vi "Pomiar charakterystyk tranzystora.vi"() -> ()   [LabVIEW 2023]
uses:
  states ilosc charakterystyk type def.ctl
  Typedef.ctl
  Open_device_2018.llb/Select_Instr.ctl
  <vilib>/Analysis/1siggen.llb/Ramp Pattern by Samples.vi
  <vilib>/Utility/file.llb/Write Delimited Spreadsheet (DBL).vi
  <vilib>/Analysis/NI_AALBase.lvlib
panel:
  in  "Zatwierdz":bool
  out "Moc 3":dbl[](array[numeric])
  out "Ic 3":dbl[](array[numeric])
  out "Uce 3":dbl[](array[numeric])
  out "XY Graph":cluster{dbl[], dbl[]}[](graph)=[{[1.0, 2.0, 4.0], [2.0, 1.0, 0.0]}, {[0.5, 1.5, 3.5], [3.0, 4.0, 2.0]}]
  out "Ic 2":dbl[](array[numeric])
  out "Moc 2":dbl[](array[numeric])
  out "Uce 2":dbl[](array[numeric])
  out "Samples 3":dbl[](array[numeric])
  out "Samples 2":dbl[](array[numeric])
  out "Samples":dbl[](array[numeric])
  in  "Maksymalne napiecie zasilania 3":i32=30
  in  "Maksymalne napiecie zasilania 2":i32=30
  in  "Maksymalne napiecie zasilania":i32=30
  in  "Ilosc punktow pomiarowych 3":i32=60
  in  "Ilosc punktow pomiarowych 2":i32=60
  in  "Ilosc punktow pomiarowych":i32=60
  out "Moc":dbl[](array[numeric])
  out "Uce":dbl[](array[numeric])
  out "Ic":dbl[](array[numeric])
  in  "Wybor operacji po pomiarze":enum16{"Exit", "Eksportuj do pliku"}(ring)
  in  "Maksymalna moc tranzystora 3":dbl(knob) scale=0.0..0.8
  in  "Maksymalna moc tranzystora 2":dbl(knob) scale=0.0..0.8
  in  "OK":bool
  out "Dzialanie programu":string
  in  "Zakoncz program":bool
  in  "Maksymalna moc tranzystora":dbl(knob) scale=0.0..0.8
  in  "Prad bazy 3":enum16{"100uA", "200uA", "300uA"}(ring)=enum."300uA"
  in  "Prad bazy 2":enum16{"100uA", "200uA", "300uA"}(ring)=enum."200uA"
  in  "Prad bazy":enum16{"100uA", "200uA", "300uA"}(ring)
  in  "Ilosc charakterystyk":T1
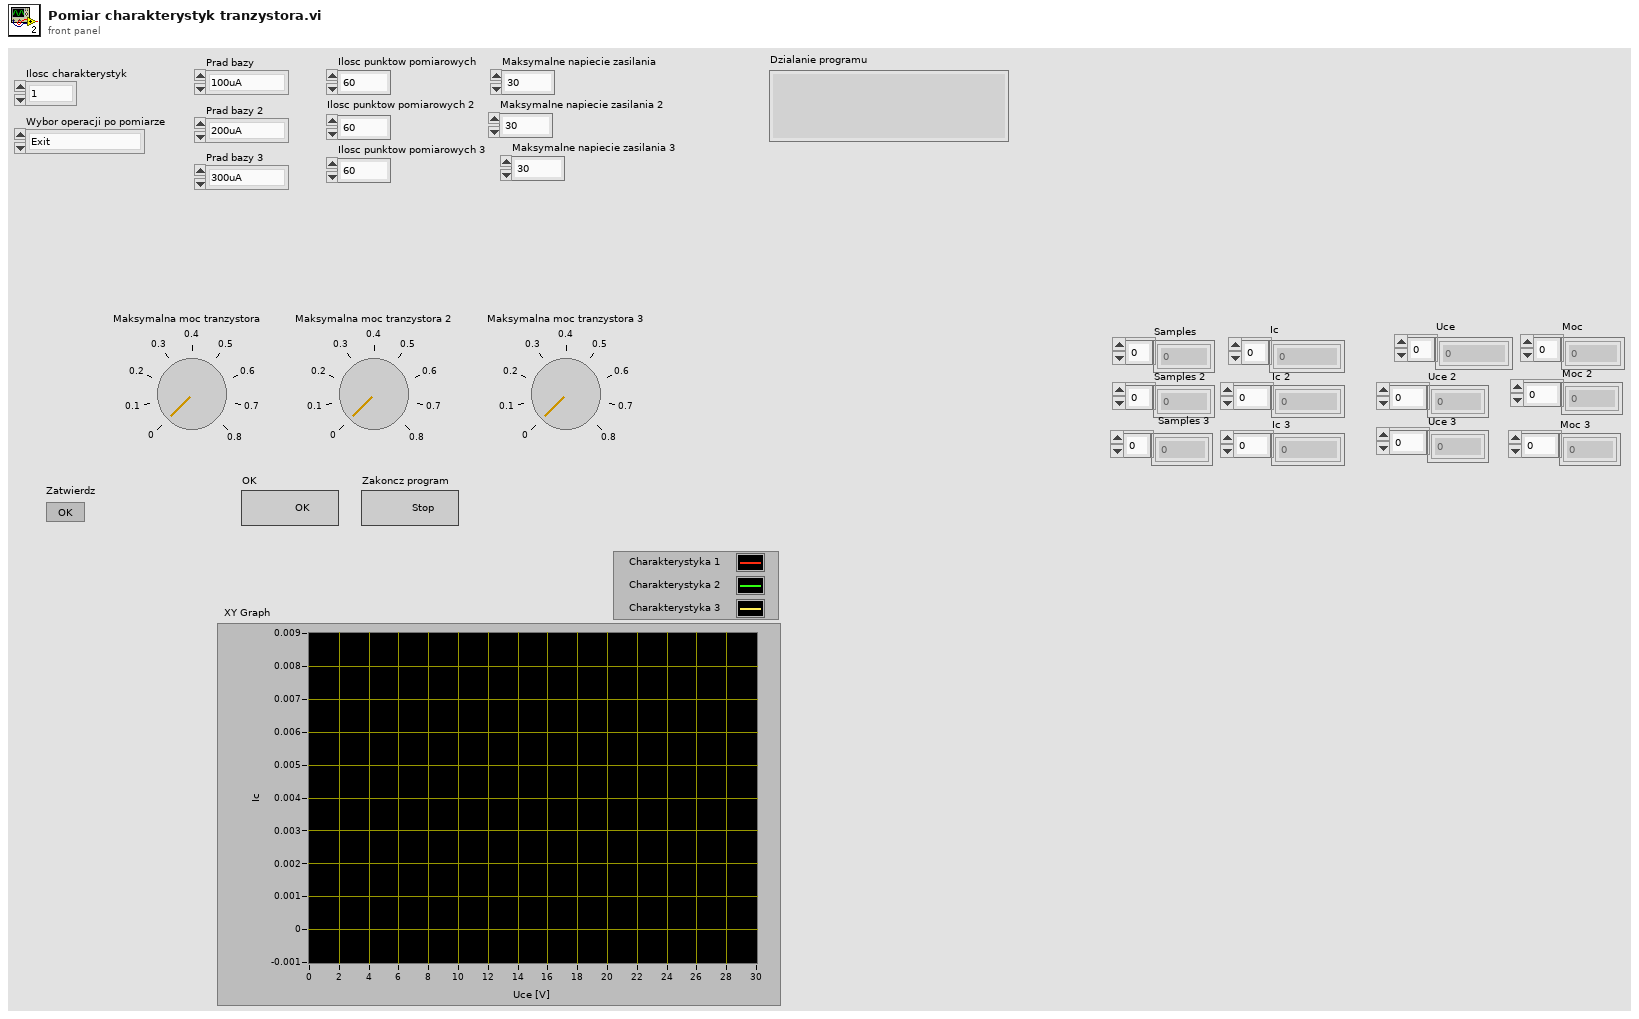
[diagram p1: front panel]
types:
  T1 = typedef "states ilosc charakterystyk type def.ctl" = enum16{"1", "2", "3"}
  T2 = typedef "Typedef.ctl" = enum16{"init", "idle", "Pomiar", "Po pomiarze", "Eksportuj do pliku", "Exit"}
  T3 = typedef "Select_Instr.ctl" = string
  T4 = cluster{"Zasilacz BM572":refnum<visa-resource-name>, "Komutator L201":refnum<visa-resource-name>, "Multimetr V553":refnum<visa-resource-name>}
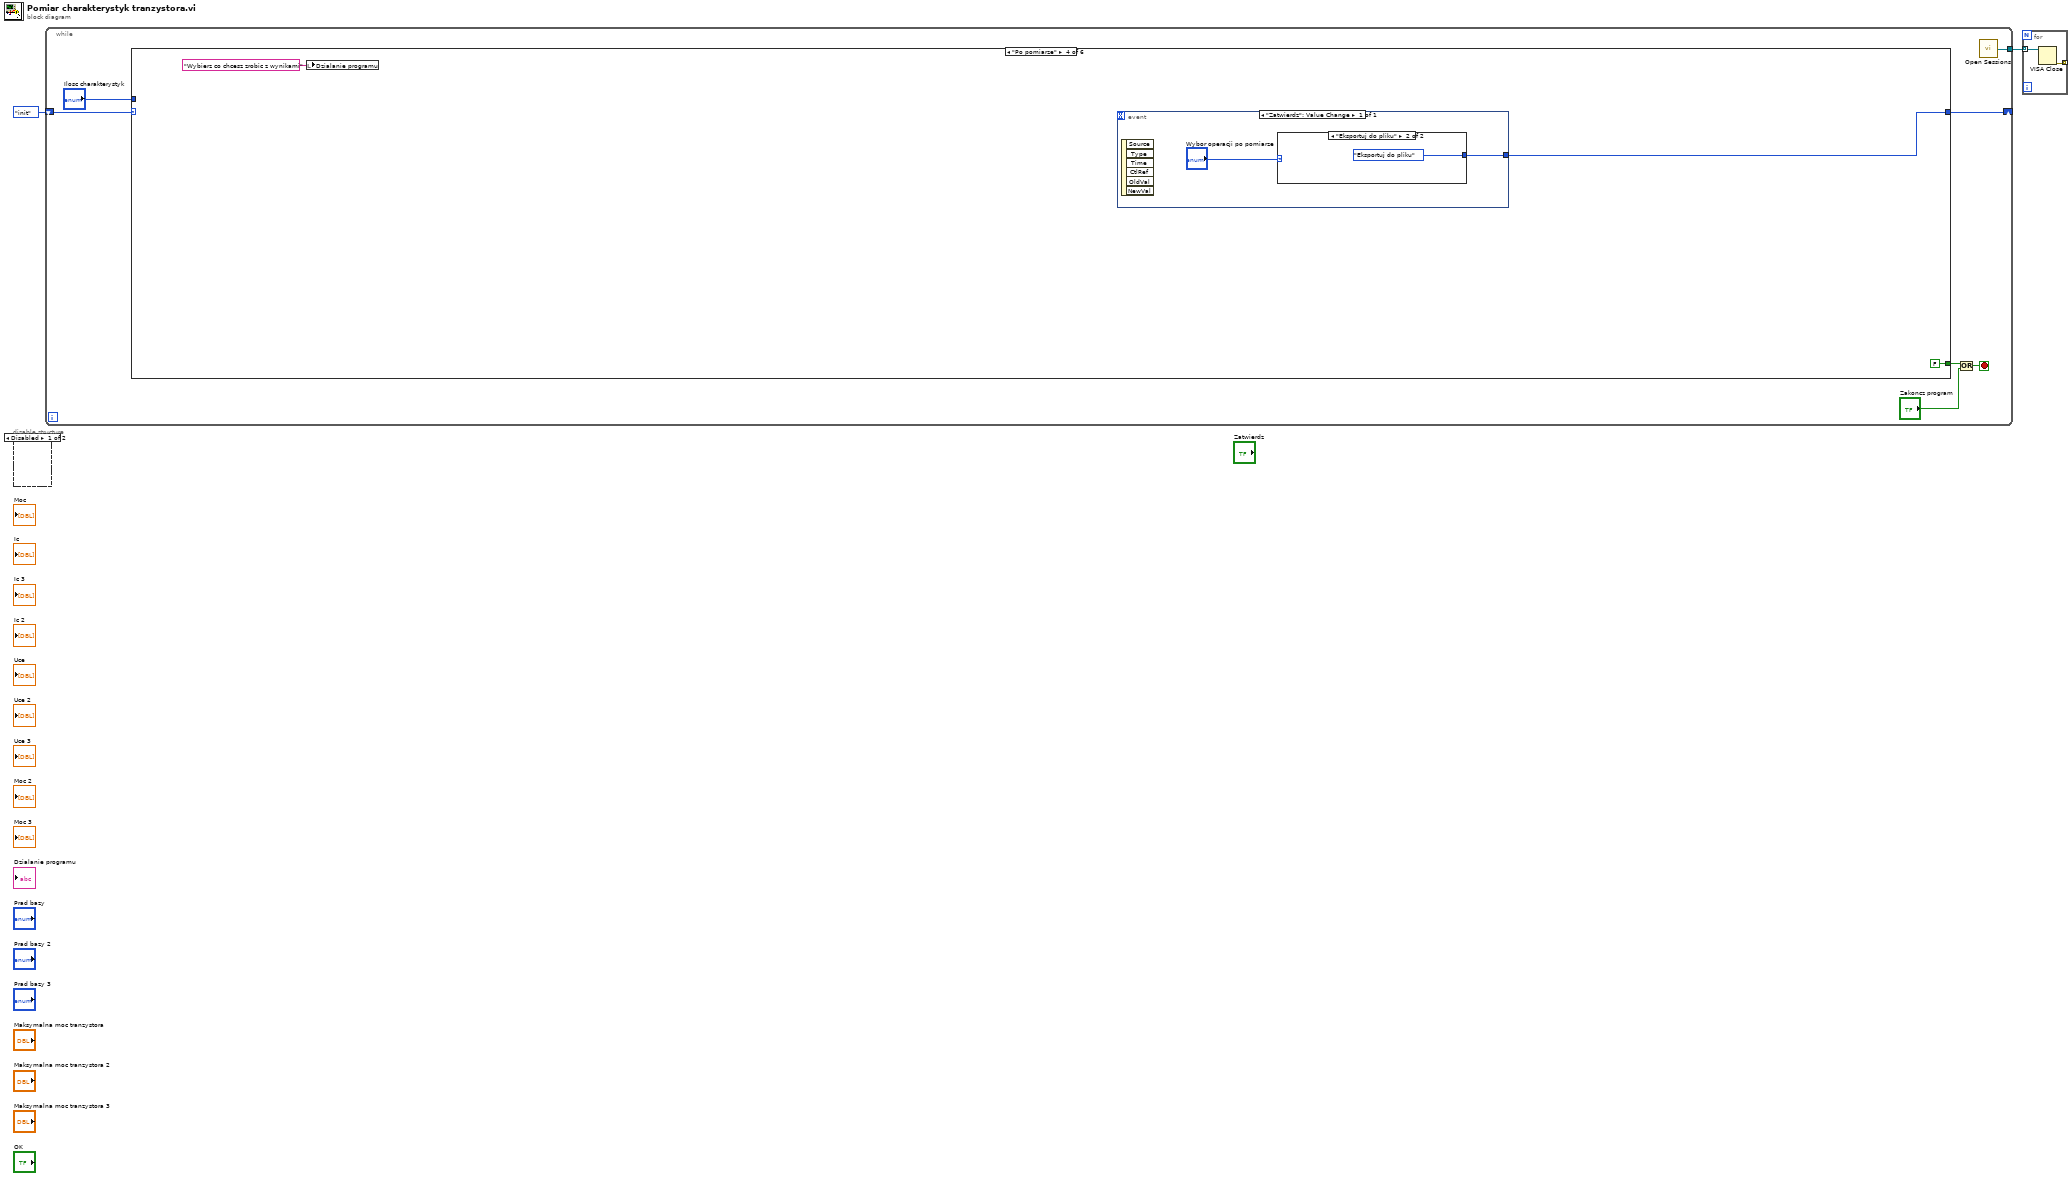
[diagram p0: block diagram]
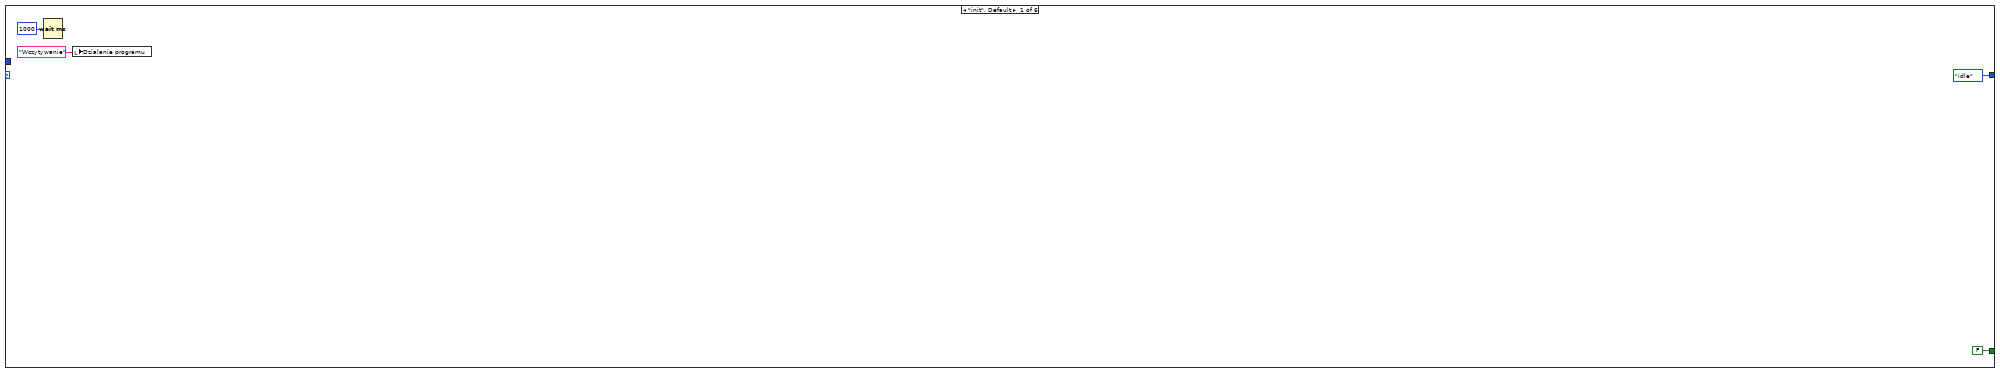
[diagram p3: hidden frame]
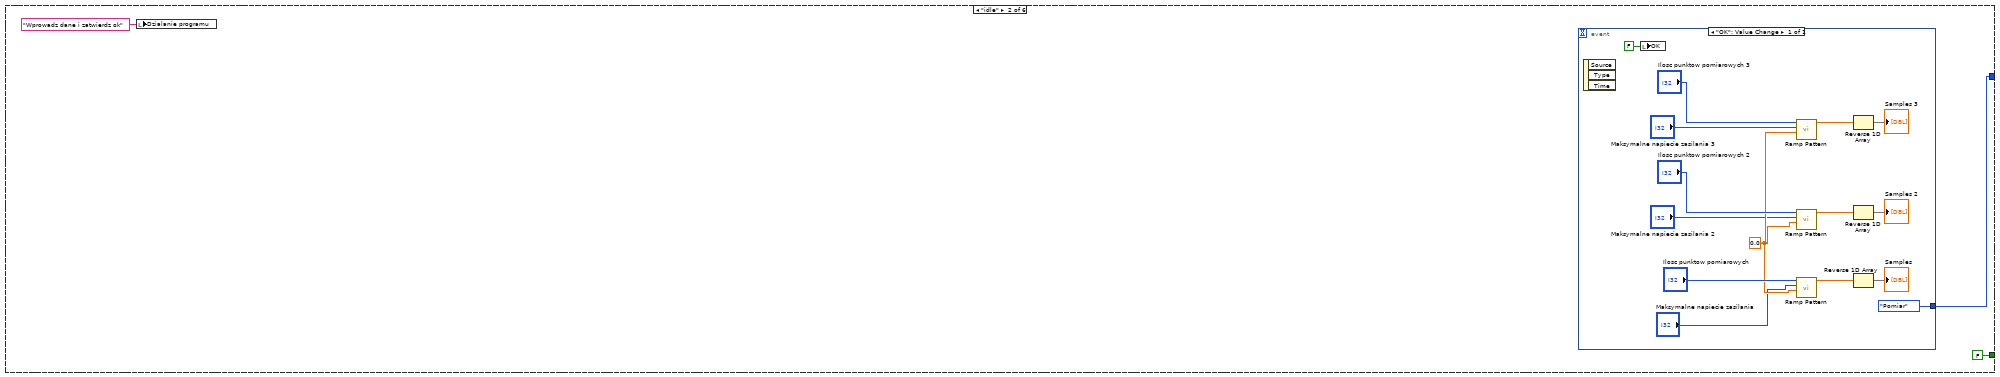
[diagram p4: hidden frame]
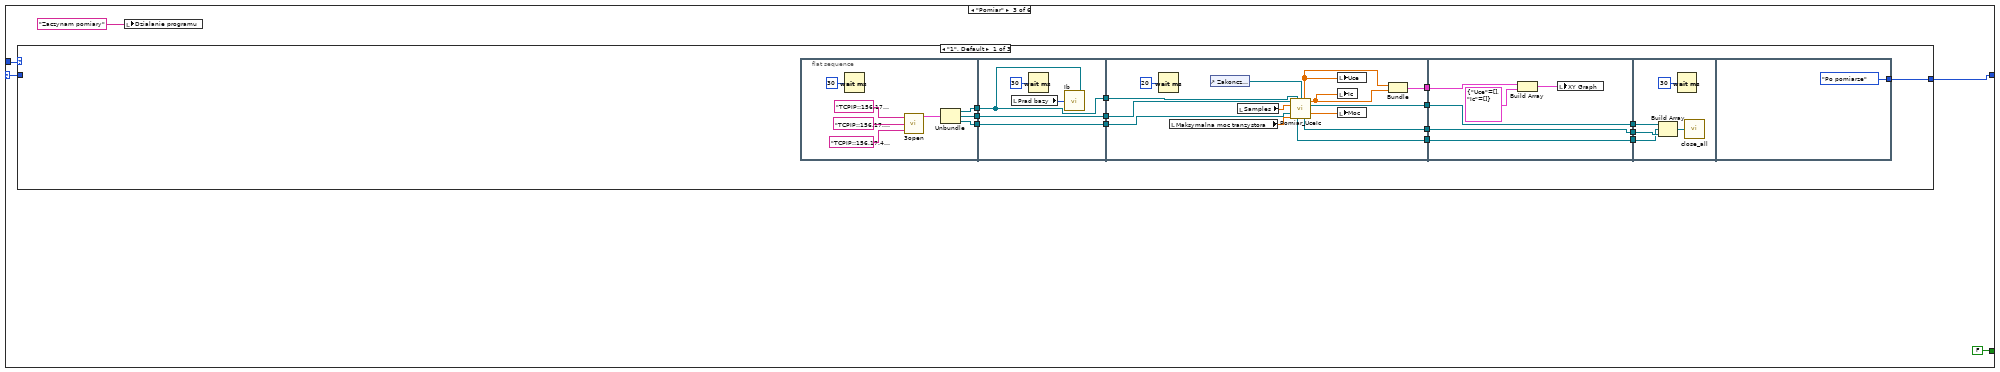
[diagram p5: hidden frame]
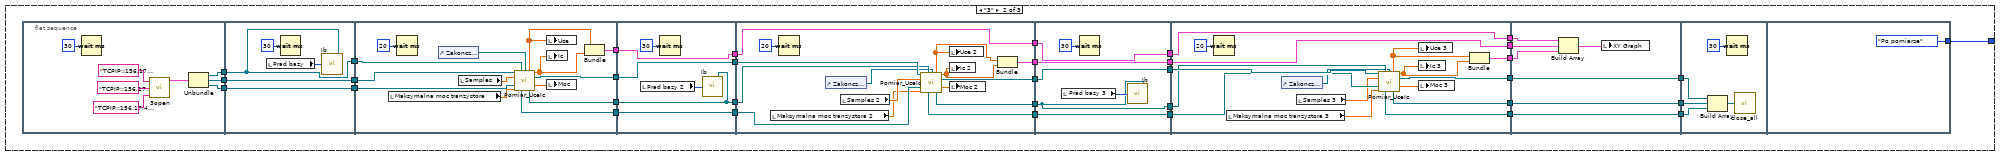
[diagram p6: hidden frame]
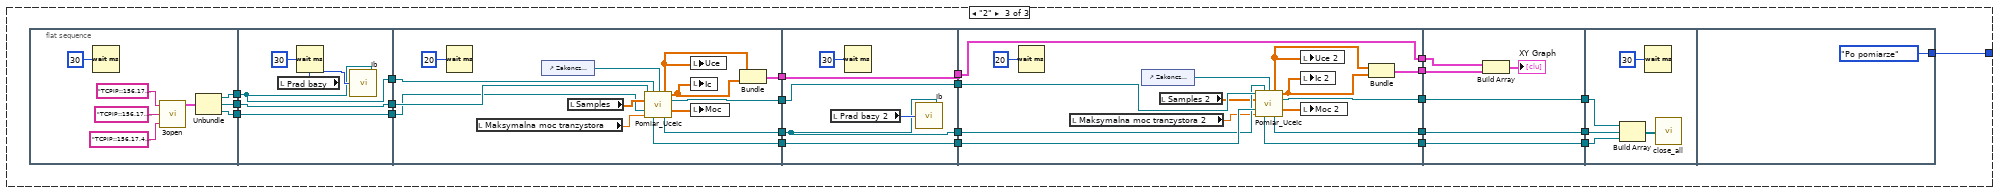
[diagram p7: hidden frame]
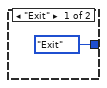
[diagram p8: hidden frame]
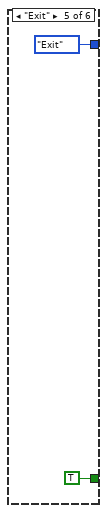
[diagram p9: hidden frame]
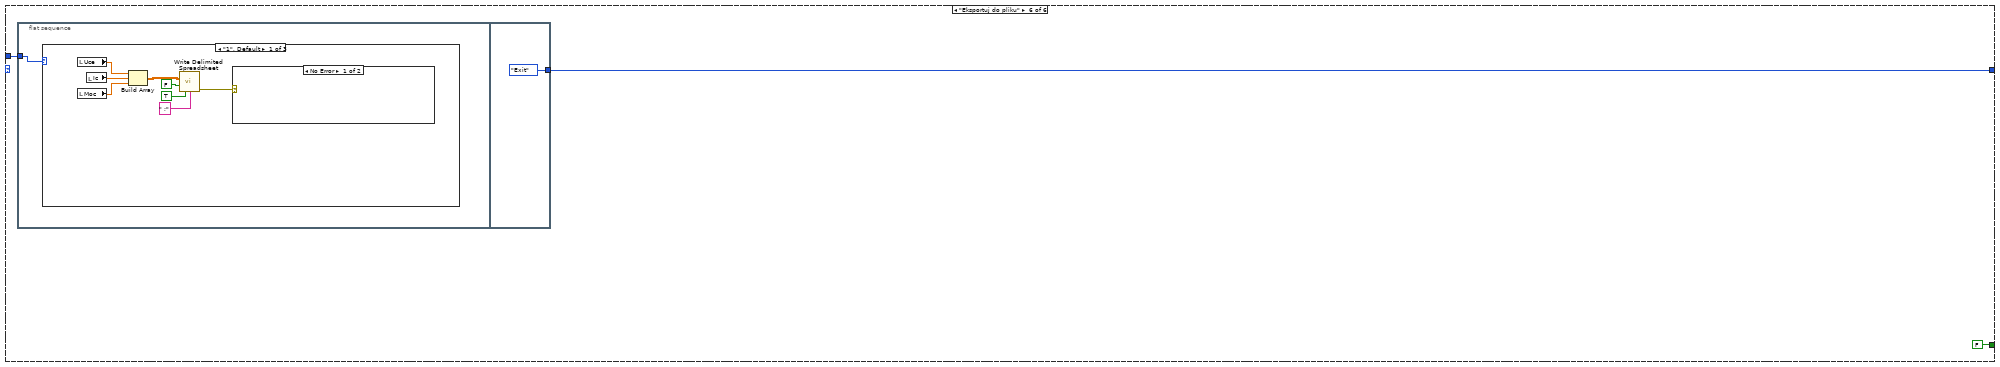
[diagram p10: hidden frame]
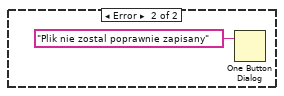
[diagram p11: hidden frame]
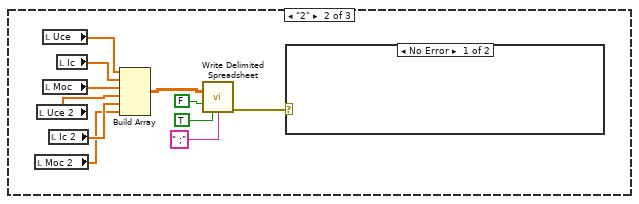
[diagram p12: hidden frame]
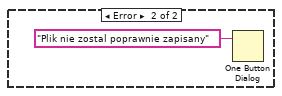
[diagram p13: hidden frame]
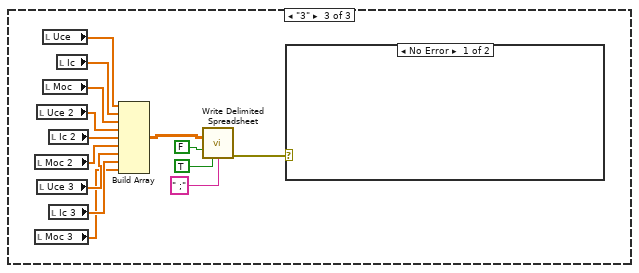
[diagram p14: hidden frame]
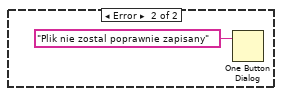
[diagram p15: hidden frame]
diagram:
  n1 = disable-structure shown="Disabled" {
    frame Disabled {
    }
    frame Enabled {
    }
  }
  n2 = while {
    shift-right: [w8] -> _
    shift-left: Typedef."init" -> [w9]
    tunnel: [w3] -> w1
    stop <- w4 stop-if-true
    n3 = case shown="\"Po pomiarze\"" w9 {
      selector: w9 -> [_ _ w32 _ _ _]
      tunnel: [Typedef."idle" w15 w34 w292 Typedef."Exit" w302] -> w8
      tunnel: "Ilosc charakterystyk" -> [_ _ w36 _ _ w301]
      tunnel: [FALSE FALSE FALSE FALSE TRUE FALSE] -> w5
      frame "init", Default {
        n4 = Wait (ms)(milliseconds to wait=u32 1000) -> ()  [unwired: 1 out]
        n5 = local write "Dzialanie programu"("Wczytywanie") -> ()
      }
      frame "idle" {
        n6 = local write "Dzialanie programu"("Wprowadz dane i zatwierdz ok") -> ()
        n7 = event shown="[0] \"OK\": Value Change" {
          selector: _ -> [_]
          dyn-events: _ -> [_]
          timeout: _ -> [_]
          tunnel: [Typedef."Pomiar"] -> w15
          event "OK": Value Change {
            w27 = 0.0 ("end")
            n8 = event-data() -> ()  [unwired: 1 in, 3 out]
            n9 = local write "OK"(FALSE ("OK")) -> ()
            n10 = call-poly <vilib>:"Ramp Pattern.vi"("start"=w27, "end"="Maksymalne napiecie zasilania 3", "samples"="Ilosc punktow pomiarowych 3") -> ("Ramp Pattern"=w22:dbl[])  [unwired: 7 in, 1 out]
            n11 = call-poly <vilib>:"Ramp Pattern.vi"("start"=w27, "end"="Maksymalne napiecie zasilania 2", "samples"="Ilosc punktow pomiarowych 2") -> ("Ramp Pattern"=w21:dbl[])  [unwired: 7 in, 1 out]
            n12 = call-poly <vilib>:"Ramp Pattern.vi"("start"=w27, "end"="Maksymalne napiecie zasilania", "samples"="Ilosc punktow pomiarowych") -> ("Ramp Pattern"=w23:dbl[])  [unwired: 7 in, 1 out]
            n13 = Reverse 1D Array(array=w22) -> (reversed array=→"Samples 3":dbl[])
            n14 = Reverse 1D Array(array=w21) -> (reversed array=→"Samples 2":dbl[])
            n15 = Reverse 1D Array(array=w23) -> (reversed array=→"Samples":dbl[])
          }
        }
      }
      frame "Pomiar" {
        n16 = case shown="\"1\", Default" w36 {
          tunnel: [w50 w90 w208] -> w34
          tunnel: w32 -> [_ _ _]
          frame "1", Default {
            n17 = flat-sequence {
              tunnel: [w53] -> w48
              tunnel: [w52] -> w46
              tunnel: [w51] -> w44
              tunnel: [w59] -> w49
              tunnel: w48 -> [w59]
              tunnel: [w62] -> w47
              tunnel: w46 -> [w62]
              tunnel: [w61] -> w45
              tunnel: w44 -> [w61]
              tunnel: w49 -> [w74]
              tunnel: w47 -> [w73]
              tunnel: w45 -> [w72]
              tunnel: [w71] -> w43
              tunnel: [w70] -> w41
              tunnel: [w69] -> w39
              tunnel: [w68] -> w37
              tunnel: w43 -> [w83]
              tunnel: [w83] -> w42
              tunnel: w41 -> [w82]
              tunnel: [w82] -> w40
              tunnel: w39 -> [w81]
              tunnel: [w81] -> w38
              tunnel: w37 -> [w80]
              tunnel: w42 -> [w87]
              tunnel: w40 -> [w86]
              tunnel: w38 -> [w85]
              tunnel: [Typedef."Po pomiarze"] -> w50
              frame #0 {
                n18 = Wait (ms)(milliseconds to wait=u32 30) -> ()  [unwired: 1 out]
                n19 = call "3open.vi"("Zasilacz BM572"=T3 "TCPIP::156.17.45.35::inst18::INSTR" ("Select_Instrument"), "Komutator L201"=T3 "TCPIP::156.17.45.35::inst19::INSTR" ("Select_Instrument"), "Multimetr V553"=T3 "TCPIP::156.17.45.35::inst21::INSTR" ("Select_Instrument")) -> ("InstrCluster"=w54:T4)  [unwired: 1 in, 3 out]
                n20 = Unbundle(w54) -> ("Zasilacz BM572"=w53:refnum<visa-resource-name>, "Komutator L201"=w52:refnum<visa-resource-name>, "Multimetr V553"=w51:refnum<visa-resource-name>)
              }
              frame #1 {
                n21 = local read "Prad bazy"() -> (w60:enum16{"100uA", "200uA", "300uA"})
                n22 = Wait (ms)(milliseconds to wait=u32 30) -> ()  [unwired: 1 out]
                n23 = call "Ib.vi"("Case"=w60, "Zasilacz BM572"=w59) -> ()  [unwired: 1 out]
              }
              frame #2 {
                n24 = Wait (ms)(milliseconds to wait=u32 20) -> ()  [unwired: 1 out]
                n25 = local read "Maksymalna moc tranzystora"() -> (w75:dbl)
                n26 = control-ref of="Zakoncz program"() -> (w64:refnum<vi>)
                n27 = local read "Samples"() -> (w76:dbl[])
                n28 = call "Pomiar_UceIc.vi"("Komutator L201"=w73, "Zasilacz BM572"=w74, "STOP"=w64, "Samples"=w76, "Multimetr V553"=w72, "Maksymalna moc tranzystora"=w75) -> ("Uce"=w67:dbl[], "Ic"=w66:dbl[], "Komutator L201 out"=w69:refnum<visa-resource-name>, "Moc [W]"=w65:dbl[], "Multimetr V553 out"=w70:refnum<visa-resource-name>, "Zasilacz BM572 out"=w71:refnum<visa-resource-name>)  [unwired: 3 in, 1 out]
                n29 = local write "Uce"(w67) -> ()
                n30 = local write "Ic"(w66) -> ()
                n31 = local write "Moc"(w65) -> ()
                n32 = Bundle("Uce"=w67, "Ic"=w66) -> (w68:cluster{"Uce":dbl[], "Ic":dbl[]})  [unwired: 1 in]
              }
              frame #3 {
                n33 = Build Array(w80, cluster{"Uce":dbl[], "Ic":dbl[]} {"Uce"=[], "Ic"=[]} ("element")) -> (w79:cluster{"Uce":dbl[], "Ic":dbl[]}[])
                n34 = local write "XY Graph"(w79) -> ()
              }
              frame #4 {
                n35 = Build Array(w85, w86, w87) -> (w84:refnum<visa-resource-name>[])
                n36 = Wait (ms)(milliseconds to wait=u32 30) -> ()  [unwired: 1 out]
                n37 = call "close_all.vi"("OpenRes"=w84) -> ()  [unwired: 1 out]
              }
              frame #5 {
              }
            }
          }
          frame "3" {
            n38 = flat-sequence {
              tunnel: [w126] -> w123
              tunnel: [w125] -> w122
              tunnel: [w124] -> w121
              tunnel: [w132] -> w120
              tunnel: w123 -> [w132]
              tunnel: [w135] -> w119
              tunnel: w122 -> [w135]
              tunnel: [w134] -> w118
              tunnel: w121 -> [w134]
              tunnel: w120 -> [w147]
              tunnel: w119 -> [w146]
              tunnel: w118 -> [w145]
              tunnel: [w144] -> w117
              tunnel: [w143] -> w116
              tunnel: [w142] -> w115
              tunnel: [w141] -> w114
              tunnel: w117 -> [w152]
              tunnel: [w152] -> w113
              tunnel: w116 -> [w156]
              tunnel: [w156] -> w112
              tunnel: w115 -> [w155]
              tunnel: [w155] -> w111
              tunnel: w114 -> [w154]
              tunnel: [w154] -> w110
              tunnel: w113 -> [w169]
              tunnel: w112 -> [w170]
              tunnel: w111 -> [w171]
              tunnel: w110 -> [w163]
              tunnel: [w166] -> w107
              tunnel: [w165] -> w105
              tunnel: [w164] -> w103
              tunnel: [w163] -> w101
              tunnel: [w158] -> w99
              tunnel: w107 -> [w178]
              tunnel: [w178] -> w106
              tunnel: w105 -> [w172]
              tunnel: [w172] -> w104
              tunnel: w103 -> [w177]
              tunnel: [w177] -> w102
              tunnel: w101 -> [w176]
              tunnel: [w176] -> w100
              tunnel: w99 -> [w175]
              tunnel: [w175] -> w98
              tunnel: w106 -> [w192]
              tunnel: w104 -> [w190]
              tunnel: w102 -> [w191]
              tunnel: w100 -> [w194]
              tunnel: [w194] -> w109
              tunnel: w98 -> [w193]
              tunnel: [w193] -> w108
              tunnel: [w187] -> w96
              tunnel: [w186] -> w94
              tunnel: [w185] -> w92
              tunnel: [w181] -> w91
              tunnel: w109 -> [w201]
              tunnel: w108 -> [w200]
              tunnel: [w198] -> w97
              tunnel: w96 -> [w198]
              tunnel: [w197] -> w95
              tunnel: w94 -> [w197]
              tunnel: [w196] -> w93
              tunnel: w92 -> [w196]
              tunnel: w91 -> [w195]
              tunnel: w97 -> [w204]
              tunnel: w95 -> [w203]
              tunnel: w93 -> [w202]
              tunnel: [Typedef."Po pomiarze"] -> w90
              frame #0 {
                n39 = Wait (ms)(milliseconds to wait=u32 30) -> ()  [unwired: 1 out]
                n40 = call "3open.vi"("Zasilacz BM572"=T3 "TCPIP::156.17.45.35::inst18::INSTR" ("Select_Instrument"), "Komutator L201"=T3 "TCPIP::156.17.45.35::inst19::INSTR" ("Select_Instrument"), "Multimetr V553"=T3 "TCPIP::156.17.45.35::inst21::INSTR" ("Select_Instrument")) -> ("InstrCluster"=w127:T4)  [unwired: 1 in, 3 out]
                n41 = Unbundle(w127) -> ("Zasilacz BM572"=w126:refnum<visa-resource-name>, "Komutator L201"=w125:refnum<visa-resource-name>, "Multimetr V553"=w124:refnum<visa-resource-name>)
              }
              frame #1 {
                n42 = local read "Prad bazy"() -> (w133:enum16{"100uA", "200uA", "300uA"})
                n43 = Wait (ms)(milliseconds to wait=u32 30) -> ()  [unwired: 1 out]
                n44 = call "Ib.vi"("Case"=w133, "Zasilacz BM572"=w132) -> ()  [unwired: 1 out]
              }
              frame #2 {
                n45 = local read "Maksymalna moc tranzystora"() -> (w148:dbl)
                n46 = Wait (ms)(milliseconds to wait=u32 20) -> ()  [unwired: 1 out]
                n47 = control-ref of="Zakoncz program"() -> (w137:refnum<vi>)
                n48 = local read "Samples"() -> (w149:dbl[])
                n49 = call "Pomiar_UceIc.vi"("Komutator L201"=w146, "Zasilacz BM572"=w147, "STOP"=w137, "Samples"=w149, "Multimetr V553"=w145, "Maksymalna moc tranzystora"=w148) -> ("Uce"=w140:dbl[], "Ic"=w139:dbl[], "Komutator L201 out"=w142:refnum<visa-resource-name>, "Moc [W]"=w138:dbl[], "Multimetr V553 out"=w143:refnum<visa-resource-name>, "Zasilacz BM572 out"=w144:refnum<visa-resource-name>)  [unwired: 3 in, 1 out]
                n50 = local write "Uce"(w140) -> ()
                n51 = local write "Ic"(w139) -> ()
                n52 = local write "Moc"(w138) -> ()
                n53 = Bundle("Uce"=w140, "Ic"=w139) -> (w141:cluster{"Uce":dbl[], "Ic":dbl[]})  [unwired: 1 in]
              }
              frame #3 {
                n54 = local read "Prad bazy 2"() -> (w153:enum16{"100uA", "200uA", "300uA"})
                n55 = Wait (ms)(milliseconds to wait=u32 30) -> ()  [unwired: 1 out]
                n56 = call "Ib.vi"("Case"=w153, "Zasilacz BM572"=w152) -> ()  [unwired: 1 out]
              }
              frame #4 {
                n57 = local read "Maksymalna moc tranzystora 2"() -> (w167:dbl)
                n58 = Wait (ms)(milliseconds to wait=u32 20) -> ()  [unwired: 1 out]
                n59 = control-ref of="Zakoncz program"() -> (w157:refnum<vi>)
                n60 = local read "Samples 2"() -> (w168:dbl[])
                n61 = call "Pomiar_UceIc.vi"("Komutator L201"=w171, "Zasilacz BM572"=w169, "STOP"=w157, "Samples"=w168, "Multimetr V553"=w170, "Maksymalna moc tranzystora"=w167) -> ("Uce"=w160:dbl[], "Ic"=w159:dbl[], "Komutator L201 out"=w166:refnum<visa-resource-name>, "Moc [W]"=w161:dbl[], "Multimetr V553 out"=w164:refnum<visa-resource-name>, "Zasilacz BM572 out"=w165:refnum<visa-resource-name>)  [unwired: 3 in, 1 out]
                n62 = local write "Uce 2"(w160) -> ()
                n63 = local write "Ic 2"(w159) -> ()
                n64 = local write "Moc 2"(w161) -> ()
                n65 = Bundle("Uce"=w160, "Ic"=w159) -> (w158:cluster{"Uce":dbl[], "Ic":dbl[]})  [unwired: 1 in]
              }
              frame #5 {
                n66 = local read "Prad bazy 3"() -> (w173:enum16{"100uA", "200uA", "300uA"})
                n67 = Wait (ms)(milliseconds to wait=u32 30) -> ()  [unwired: 1 out]
                n68 = call "Ib.vi"("Case"=w173, "Zasilacz BM572"=w172) -> ()  [unwired: 1 out]
              }
              frame #6 {
                n69 = Wait (ms)(milliseconds to wait=u32 20) -> ()  [unwired: 1 out]
                n70 = local read "Maksymalna moc tranzystora 3"() -> (w189:dbl)
                n71 = control-ref of="Zakoncz program"() -> (w179:refnum<vi>)
                n72 = local read "Samples 3"() -> (w188:dbl[])
                n73 = call "Pomiar_UceIc.vi"("Komutator L201"=w192, "Zasilacz BM572"=w190, "STOP"=w179, "Samples"=w188, "Multimetr V553"=w191, "Maksymalna moc tranzystora"=w189) -> ("Uce"=w183:dbl[], "Ic"=w182:dbl[], "Komutator L201 out"=w187:refnum<visa-resource-name>, "Moc [W]"=w184:dbl[], "Multimetr V553 out"=w185:refnum<visa-resource-name>, "Zasilacz BM572 out"=w186:refnum<visa-resource-name>)  [unwired: 3 in, 1 out]
                n74 = local write "Uce 3"(w183) -> ()
                n75 = local write "Ic 3"(w182) -> ()
                n76 = local write "Moc 3"(w184) -> ()
                n77 = Bundle("Uce"=w183, "Ic"=w182) -> (w181:cluster{"Uce":dbl[], "Ic":dbl[]})  [unwired: 1 in]
              }
              frame #7 {
                n78 = Build Array(w201, w200, w195) -> (w199:cluster{"Uce":dbl[], "Ic":dbl[]}[])
                n79 = local write "XY Graph"(w199) -> ()
              }
              frame #8 {
                n80 = Build Array(w204, w203, w202) -> (w205:refnum<visa-resource-name>[])
                n81 = Wait (ms)(milliseconds to wait=u32 30) -> ()  [unwired: 1 out]
                n82 = call "close_all.vi"("OpenRes"=w205) -> ()  [unwired: 1 out]
              }
              frame #9 {
              }
            }
          }
          frame "2" {
            n83 = flat-sequence {
              tunnel: [w233] -> w230
              tunnel: [w232] -> w229
              tunnel: [w231] -> w228
              tunnel: [w239] -> w227
              tunnel: w230 -> [w239]
              tunnel: [w242] -> w226
              tunnel: w229 -> [w242]
              tunnel: [w241] -> w225
              tunnel: w228 -> [w241]
              tunnel: w227 -> [w254]
              tunnel: w226 -> [w253]
              tunnel: w225 -> [w252]
              tunnel: [w251] -> w217
              tunnel: [w250] -> w215
              tunnel: [w249] -> w213
              tunnel: [w248] -> w211
              tunnel: w217 -> [w259]
              tunnel: [w259] -> w216
              tunnel: w215 -> [w263]
              tunnel: [w263] -> w214
              tunnel: w213 -> [w262]
              tunnel: [w262] -> w212
              tunnel: w211 -> [w261]
              tunnel: [w261] -> w210
              tunnel: w216 -> [w276]
              tunnel: w214 -> [w277]
              tunnel: w212 -> [w278]
              tunnel: w210 -> [w270]
              tunnel: [w273] -> w223
              tunnel: [w272] -> w221
              tunnel: [w271] -> w219
              tunnel: [w270] -> w218
              tunnel: [w265] -> w209
              tunnel: [w284] -> w224
              tunnel: w223 -> [w284]
              tunnel: [w283] -> w222
              tunnel: w221 -> [w283]
              tunnel: [w282] -> w220
              tunnel: w219 -> [w282]
              tunnel: w218 -> [w281]
              tunnel: w209 -> [w280]
              tunnel: w224 -> [w287]
              tunnel: w222 -> [w286]
              tunnel: w220 -> [w285]
              tunnel: [Typedef."Po pomiarze"] -> w208
              frame #0 {
                n84 = Wait (ms)(milliseconds to wait=u32 30) -> ()  [unwired: 1 out]
                n85 = call "3open.vi"("Zasilacz BM572"=T3 "TCPIP::156.17.45.35::inst18::INSTR" ("Select_Instrument"), "Komutator L201"=T3 "TCPIP::156.17.45.35::inst19::INSTR" ("Select_Instrument"), "Multimetr V553"=T3 "TCPIP::156.17.45.35::inst21::INSTR" ("Select_Instrument")) -> ("InstrCluster"=w234:T4)  [unwired: 1 in, 3 out]
                n86 = Unbundle(w234) -> ("Zasilacz BM572"=w233:refnum<visa-resource-name>, "Komutator L201"=w232:refnum<visa-resource-name>, "Multimetr V553"=w231:refnum<visa-resource-name>)
              }
              frame #1 {
                n87 = local read "Prad bazy"() -> (w240:enum16{"100uA", "200uA", "300uA"})
                n88 = Wait (ms)(milliseconds to wait=u32 30) -> ()  [unwired: 1 out]
                n89 = call "Ib.vi"("Case"=w240, "Zasilacz BM572"=w239) -> ()  [unwired: 1 out]
              }
              frame #2 {
                n90 = Wait (ms)(milliseconds to wait=u32 20) -> ()  [unwired: 1 out]
                n91 = local read "Maksymalna moc tranzystora"() -> (w255:dbl)
                n92 = control-ref of="Zakoncz program"() -> (w244:refnum<vi>)
                n93 = local read "Samples"() -> (w256:dbl[])
                n94 = call "Pomiar_UceIc.vi"("Komutator L201"=w253, "Zasilacz BM572"=w254, "STOP"=w244, "Samples"=w256, "Multimetr V553"=w252, "Maksymalna moc tranzystora"=w255) -> ("Uce"=w247:dbl[], "Ic"=w246:dbl[], "Komutator L201 out"=w249:refnum<visa-resource-name>, "Moc [W]"=w245:dbl[], "Multimetr V553 out"=w250:refnum<visa-resource-name>, "Zasilacz BM572 out"=w251:refnum<visa-resource-name>)  [unwired: 3 in, 1 out]
                n95 = local write "Uce"(w247) -> ()
                n96 = local write "Ic"(w246) -> ()
                n97 = local write "Moc"(w245) -> ()
                n98 = Bundle("Uce"=w247, "Ic"=w246) -> (w248:cluster{"Uce":dbl[], "Ic":dbl[]})  [unwired: 1 in]
              }
              frame #3 {
                n99 = local read "Prad bazy 2"() -> (w260:enum16{"100uA", "200uA", "300uA"})
                n100 = Wait (ms)(milliseconds to wait=u32 30) -> ()  [unwired: 1 out]
                n101 = call "Ib.vi"("Case"=w260, "Zasilacz BM572"=w259) -> ()  [unwired: 1 out]
              }
              frame #4 {
                n102 = Wait (ms)(milliseconds to wait=u32 20) -> ()  [unwired: 1 out]
                n103 = local read "Maksymalna moc tranzystora 2"() -> (w274:dbl)
                n104 = control-ref of="Zakoncz program"() -> (w264:refnum<vi>)
                n105 = local read "Samples 2"() -> (w275:dbl[])
                n106 = call "Pomiar_UceIc.vi"("Komutator L201"=w278, "Zasilacz BM572"=w276, "STOP"=w264, "Samples"=w275, "Multimetr V553"=w277, "Maksymalna moc tranzystora"=w274) -> ("Uce"=w267:dbl[], "Ic"=w266:dbl[], "Komutator L201 out"=w273:refnum<visa-resource-name>, "Moc [W]"=w268:dbl[], "Multimetr V553 out"=w271:refnum<visa-resource-name>, "Zasilacz BM572 out"=w272:refnum<visa-resource-name>)  [unwired: 3 in, 1 out]
                n107 = local write "Uce 2"(w267) -> ()
                n108 = local write "Ic 2"(w266) -> ()
                n109 = local write "Moc 2"(w268) -> ()
                n110 = Bundle("Uce"=w267, "Ic"=w266) -> (w265:cluster{"Uce":dbl[], "Ic":dbl[]})  [unwired: 1 in]
              }
              frame #5 {
                n111 = Build Array(w281, w280) -> (→"XY Graph":cluster{"Uce":dbl[], "Ic":dbl[]}[])
              }
              frame #6 {
                n112 = Build Array(w287, w286, w285) -> (w288:refnum<visa-resource-name>[])
                n113 = Wait (ms)(milliseconds to wait=u32 30) -> ()  [unwired: 1 out]
                n114 = call "close_all.vi"("OpenRes"=w288) -> ()  [unwired: 1 out]
              }
              frame #7 {
              }
            }
          }
        }
        n115 = local write "Dzialanie programu"("Zaczynam pomiary") -> ()
      }
      frame "Po pomiarze" {
        n116 = local write "Dzialanie programu"("Wybierz co chcesz zrobic z wynikami") -> ()
        n117 = event shown="[0] \"Zatwierdz\": Value Change" {
          selector: _ -> [_]
          dyn-events: _ -> [_]
          timeout: _ -> [_]
          tunnel: [w295] -> w292
          event "Zatwierdz": Value Change {
            n118 = event-data() -> ()  [unwired: 1 in, 6 out]
            n119 = case shown="\"Eksportuj do pliku\"" "Wybor operacji po pomiarze" {
              tunnel: [Typedef."Exit" Typedef."Eksportuj do pliku"] -> w295
              frame "Exit" {
              }
              frame "Eksportuj do pliku" {
              }
            }
          }
        }
      }
      frame "Exit" {
      }
      frame "Eksportuj do pliku" {
        n120 = flat-sequence {
          tunnel: w301 -> [w303]
          tunnel: [Typedef."Exit"] -> w302
          frame #0 {
            n121 = case shown="\"1\", Default" w303 {
              frame "1", Default {
                n122 = local read "Uce"() -> (w308:dbl[])
                n123 = local read "Moc"() -> (w306:dbl[])
                n124 = local read "Ic"() -> (w307:dbl[])
                n125 = Build Array(w308, w307, w306) -> (w305:dbl[][])
                n126 = call-poly <vilib>:"Write Delimited Spreadsheet.vi"("2D data"=w305, "append to file? (new file:F)"=FALSE, "transpose? (no:F)"=TRUE, "delimiter (\\t)"=" ;" ("delimiter (\\t)")) -> ("error out"=w304:errorcluster)  [unwired: 10 in, 1 out]
                n127 = case shown="No Error" w304 {
                  frame No Error {
                  }
                  frame Error {
                    n128 = One Button Dialog(message="Plik nie zostal poprawnie zapisany") -> ()  [unwired: 1 in, 1 out]
                  }
                }
              }
              frame "2" {
                n129 = local read "Moc 2"() -> (w316:dbl[])
                n130 = local read "Uce 2"() -> (w318:dbl[])
                n131 = local read "Uce"() -> (w321:dbl[])
                n132 = local read "Moc"() -> (w319:dbl[])
                n133 = local read "Ic 2"() -> (w317:dbl[])
                n134 = local read "Ic"() -> (w320:dbl[])
                n135 = Build Array(w321, w320, w319, w318, w317, w316) -> (w315:dbl[][])
                n136 = call-poly <vilib>:"Write Delimited Spreadsheet.vi"("2D data"=w315, "append to file? (new file:F)"=FALSE, "transpose? (no:F)"=TRUE, "delimiter (\\t)"=" ;" ("delimiter (\\t)")) -> ("error out"=w313:errorcluster)  [unwired: 10 in, 1 out]
                n137 = case shown="No Error" w313 {
                  frame No Error {
                  }
                  frame Error {
                    n138 = One Button Dialog(message="Plik nie zostal poprawnie zapisany") -> ()  [unwired: 1 in, 1 out]
                  }
                }
              }
              frame "3" {
                n139 = local read "Moc 2"() -> (w330:dbl[])
                n140 = local read "Moc 3"() -> (w327:dbl[])
                n141 = local read "Uce 2"() -> (w332:dbl[])
                n142 = local read "Uce 3"() -> (w329:dbl[])
                n143 = local read "Uce"() -> (w335:dbl[])
                n144 = local read "Moc"() -> (w333:dbl[])
                n145 = local read "Ic 2"() -> (w331:dbl[])
                n146 = local read "Ic 3"() -> (w328:dbl[])
                n147 = local read "Ic"() -> (w334:dbl[])
                n148 = Build Array(w335, w334, w333, w332, w331, w330, w329, w328, w327) -> (w326:dbl[][])
                n149 = call-poly <vilib>:"Write Delimited Spreadsheet.vi"("2D data"=w326, "append to file? (new file:F)"=FALSE, "transpose? (no:F)"=TRUE, "delimiter (\\t)"=" ;" ("delimiter (\\t)")) -> ("error out"=w325:errorcluster)  [unwired: 10 in, 1 out]
                n150 = case shown="No Error" w325 {
                  frame No Error {
                  }
                  frame Error {
                    n151 = One Button Dialog(message="Plik nie zostal poprawnie zapisany") -> ()  [unwired: 1 in, 1 out]
                  }
                }
              }
            }
          }
          frame #1 {
          }
        }
      }
    }
    n152 = Or(x=w5, y="Zakoncz program") -> (x .or. y?=w4:bool)
    n153 = call <vilib>:"Open Sessions.vi"() -> ("Array of Refnums"=w3:refnum<visa-resource-name>[])  [unwired: 2 out]
  }
  n154 = for {
    tunnel: w1 -> [w342] mode=indexing
    tunnel: [w341] -> _ mode=indexing
    n155 = VISA Close(VISA resource name=w342) -> (error out=w341:errorcluster)  [unwired: 1 in]
  }
